vi "convertErrorCode.vi"(1 "error in":errorcluster, 2 "error code":i32) -> (0 "error out":errorcluster)   [LabVIEW 2011]
doc: "This VI converts returned error codes into text descriptions of the error."
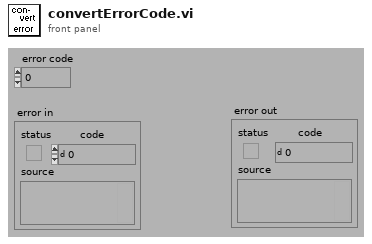
[diagram p1: front panel]
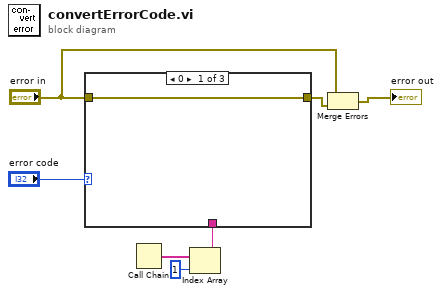
[diagram p0: block diagram]
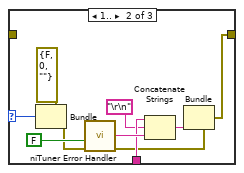
[diagram p2: hidden frame]
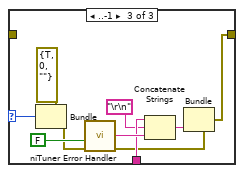
[diagram p3: hidden frame]
diagram:
  n1 = Call Chain() -> (call chain=w6:string[])
  n2 = Index Array(array=w6, index=1 ("Index")) -> (element=w4:string)
  n3 = case shown="0" "error code" {
    selector: "error code" -> [_ w9 w19]
    tunnel: [w8 w18 w28] -> w3
    tunnel: "error in" -> [w8 _ _]
    tunnel: w4 -> [_ w15 w25]
    frame 0 {
    }
    frame 1.. {
      n4 = Bundle(cluster=errorcluster {"status"=FALSE, "code"=0, "source"=""} ("error IO"), "code"=w9) -> (w10:errorcluster)  [unwired: 2 in]
      n5 = call <instrlib>:"niTuner Error Handler.vi"("error in"=w10, "pop up message?"=FALSE) -> ("error out"=w13:errorcluster, "error message"=w16:string)  [unwired: 7 in, 1 out]
      n6 = Concatenate Strings(w15, "\r\n", w16) -> (w12:string)
      n7 = Bundle(cluster=w13, "source"=w12) -> (w18:errorcluster)  [unwired: 2 in]
    }
    frame ..-1 {
      n8 = Bundle(cluster=errorcluster {"status"=TRUE, "code"=0, "source"=""} ("error IO"), "code"=w19) -> (w20:errorcluster)  [unwired: 2 in]
      n9 = call <instrlib>:"niTuner Error Handler.vi"("error in"=w20, "pop up message?"=FALSE) -> ("error out"=w23:errorcluster, "error message"=w26:string)  [unwired: 7 in, 1 out]
      n10 = Concatenate Strings(w25, "\r\n", w26) -> (w22:string)
      n11 = Bundle(cluster=w23, "source"=w22) -> (w28:errorcluster)  [unwired: 2 in]
    }
  }
  n12 = Merge Errors("error in", w3) -> (→"error out":errorcluster)
